vi "SetTilesByStringQueue.vi"(8 "error in (no error)":errorcluster, 9 "Position":T1, 10 "TileStrings":string[][](array[string]), 11 "Game in":refnum<class "Game.lvclass">) -> (0 "error out":errorcluster, 3 "Game out":refnum<class "Game.lvclass">)   [LabVIEW 2019, in "RT_Game.lvlib" / "Game.lvclass"]
uses:
  Game.lvclass
  Coordinate.ctl
  Game.lvclass/Game.ctl
  Engine/Engine.lvclass
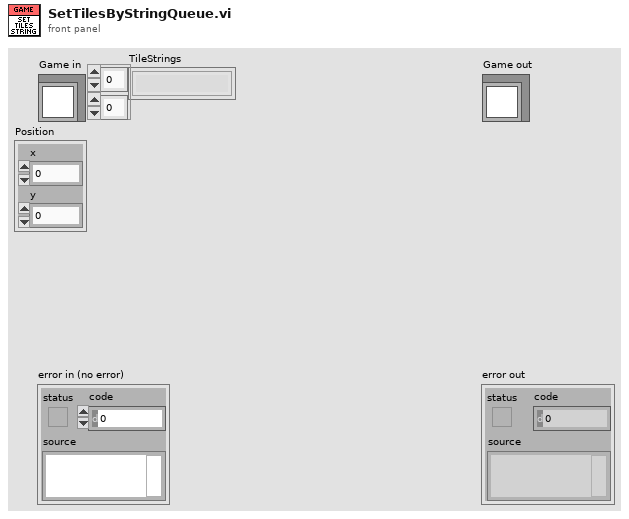
[diagram p1: front panel]
types:
  T1 = typedef "RT_Game.lvlib/Game.lvclass/Coordinate.ctl" = cluster{"x":dbl, "y":dbl}
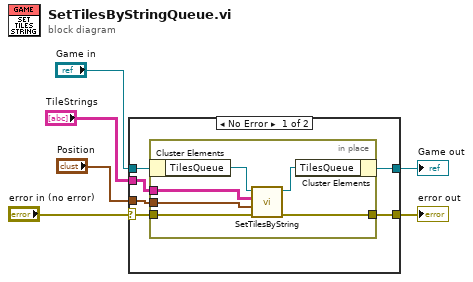
[diagram p0: block diagram]
diagram:
  n1 = case shown="No Error" "error in (no error)" {
    selector: "error in (no error)" -> [w12 w20]
    tunnel: [w11 w20] -> w5
    tunnel: [w10 w19] -> w3
    tunnel: "Game in" -> [w9 w19]
    tunnel: "Position" -> [w8 _]
    tunnel: "TileStrings" -> [w7 _]
    frame No Error {
      n2 = in-place {
        in-place-border: w12 -> [w18]
        in-place-border: [w17] -> w11
        in-place-border: w8 -> [w14]
        in-place-border: w7 -> [w13]
        n3 = in-place-cluster #1(w9) -> ("TilesQueue"=w16:refnum<queue>)
        n4 = call "SetTilesByString.vi"("error in (no error)"=w18, "Position"=w14, "TileStrings"=w13, "TilesQueue"=w16) -> ("error out"=w17:errorcluster, "TilesQueue out"=w15:refnum<queue>)  [unwired: 6 in]
        n5 = in-place-cluster #1("TilesQueue"=w15) -> (w10:refnum<class "Game.lvclass">)
      }
    }
    frame Error {
    }
  }
  "error out" <- w5
  "Game out" <- w3
